vi "Display_LookUpMapTile.vi"(1 "ActivePixel":T3, 4 "ActiveTile":T1) -> (15 "ActiveTile":T2, 18 "TilePixelOffset":i16)   [LabVIEW 2018]
uses:
  TypDefs/ActivePixel_Cluster.ctl
  TypDefs/Tile_Enum.ctl
  TypDefs/ActiveTile_Cluster.ctl
  <vilib>/rvi/DataTransferAndStorage/Container/Common/niFpgaContainerExecOnDevCompGetState.vi
  <vilib>/rvi/Emulation/niFpgaEmulationIsFPGAContextNoSignature.vi
  <vilib>/rvi/DataTransferAndStorage/Container/Common/niFpgaContainerGetUniqueNameForEmu.vi
  <vilib>/rvi/Emulation/niFpgaProcessEmulError.vi
  <vilib>/rvi/Emulation/niFpgaSctlEmulationGetInTimedLoop.vi
  <vilib>/rvi/errors/nirviReportUnexpectedCaseInternalError (U32).vi
  <vilib>/rvi/Memory/Memory_Emulation/niFpgaMemoryEmulationCacheClearOnFirstRun.vi
  <vilib>/rvi/Memory/Memory_Emulation/nirvimemoryEmulationManagerCache_MakeExclusive.vi
  <vilib>/rvi/Memory/Memory_Emulation/niFpgaMemoryEmulationValidateCache.vi
  <vilib>/rvi/Memory/Memory_Emulation/nirvimemoryEmulationManagerCache_InsertValue.vi
  <vilib>/Utility/error.llb/Clear Errors.vi
  <vilib>/rvi/Memory/Memory_Emulation/nirvimemoryEmulationManagerCache_ReleaseExclusive.vi
  <vilib>/rvi/Memory/Memory_Emulation/nirvimemoryEmulationManagerCache_GetValue.vi
  <vilib>/rvi/Memory/Memory_Emulation/nirvimemoryEmulationManagerCache_SetValue.vi
  <vilib>/rvi/Emulation/niFpgaSctlEmulationResourceMgr.vi
  <vilib>/rvi/DataTransferAndStorage/Container/XNode/niFpgaContainer.xnode
  <vilib>/rvi/Memory/Memory_Emulation/niFpgaMemoryEmulationRefIn.vi
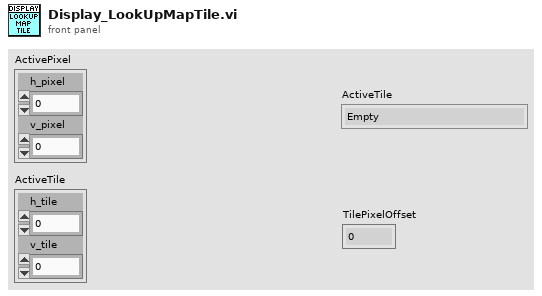
[diagram p1: front panel]
types:
  T1 = typedef "ActiveTile_Cluster.ctl" = cluster{"h_tile":i16, "v_tile":i16}
  T2 = typedef "Tile_Enum.ctl" = enum8{"Empty", "Snake1_HeadPointingUp", "Snake1_HeadPointingDown", "Snake1_HeadPoiningLeft", "Snake1_HeadPointingRight", "Snake1_DeadPointingUp", "Snake1_DeadPointingDown", "Snake1_DeadPointingLeft", "Snake1_DeadPointingRight", "Snake1_TailPointingUp", "Snake1_TailPointingDown", "Snake1_TailPointingLeft", "Snake1_TailPointingRight", "Snake1_Horizontal", "Snake1_Vertical", "Snake1_UpperLeftCorner", "Snake1_UpperRightCorner", "Snake1_LowerLeftCorner", "Snake1_LowerRightCorner", "Wall_Horizontal", "Wall_Vertical", "Wall_UpperLeftCorner", "Wall_UpperRightCorner", "Wall_LowerLeftCorner", "Wall_LowerRightCorner", "Pickup_SpeedUp", "Pickup_SlowDown", "Pickup_Banana", "Pickup_Grapes", "Pickup_Apple"}
  T3 = typedef "ActivePixel_Cluster.ctl" = cluster{"h_pixel":i16, "v_pixel":i16}
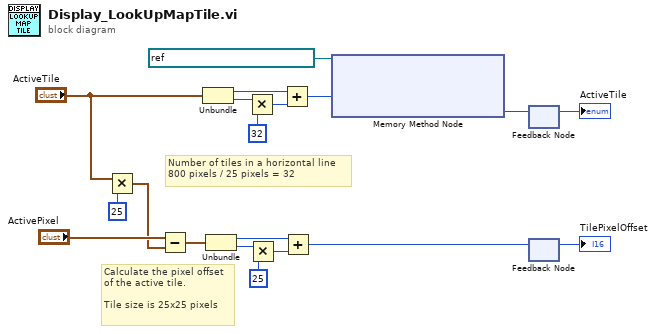
[diagram p0: block diagram]
diagram:
  # "Number of tiles in a horizontal line\n800 pixels / 25 pixels = 32"
  # "Calculate the pixel offset\nof the active tile.\n\nTile size is 25x25 pixels"
  n1 = Multiply(x="ActiveTile", y=i16 25) -> (x*y=w16:T1)
  n2 = Subtract(x="ActivePixel", y=w16) -> (x-y=w11:T3)
  n3 = Unbundle("ActiveTile") -> ("h_tile"=w3:i16, "v_tile"=w2:i16)
  n4 = Unbundle(w11) -> ("h_pixel"=w13:i16, "v_pixel"=w15:i16)
  n5 = Multiply(x=w2, y=i16 32) -> (x*y=w5:i16)
  n6 = Multiply(x=w15, y=i16 25) -> (x*y=w12:i16)
  n7 = Add(x=w3, y=w5) -> (x+y=w4:i16)
  n8 = Add(x=w13, y=w12) -> (x+y=w19:i16)
  n9 = xnode ("Memory Method Node")("Address"=w4, "Memory In"=refnum<k21> "BlockMem_FastGameMap") -> ("Data"=w7:u8)  [unwired: 1 out]
  n10 = feedback #1() -> (→"ActiveTile":u8)  [unwired: 1 in]
  n11 = feedback-in #1(w7) -> ()
  n12 = feedback #2() -> (→"TilePixelOffset":i16)  [unwired: 1 in]
  n13 = feedback-in #2(w19) -> ()
